vi "OutputDefault.vi"(6 "error in":errorcluster, 9 "Control Terminal in":refnum<class "ControlTerminal.lvclass">) -> (0 "error out":errorcluster, 3 "Control Terminal out":refnum<class "ControlTerminal.lvclass">, 4 "output default":string)   [LabVIEW 2014, in "ControlTerminal.lvclass"]
uses:
  ControlTerminal.lvclass
  Python/Parsing/Python Functions.lvlib
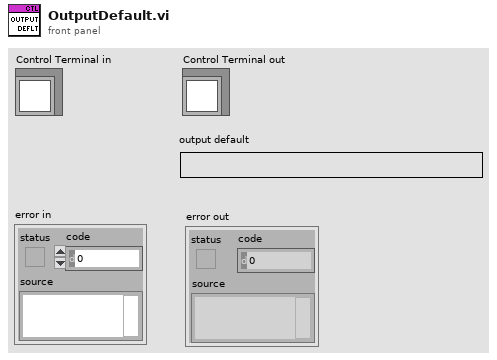
[diagram p1: front panel]
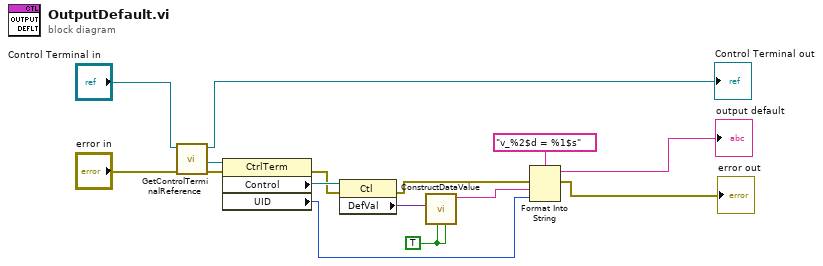
[diagram p0: block diagram]
diagram:
  w11 = TRUE ("value")
  n1 = call "GetControlTerminalReference.vi"("error in"="error in", "ControlTerminal in"="Control Terminal in") -> ("error out"=w5:errorcluster, "reference"=w4:refnum<vi>, "ControlTerminal out"=→"Control Terminal out":refnum<class "ControlTerminal.lvclass">)  [unwired: 7 in]
  n2 = property class="CtrlTerm"(reference=w4, error in=w5) -> (error out=w13:errorcluster, "Control"=w14:refnum<vi>, "UID"=w7:i32)  [unwired: 1 out]
  n3 = property class="Ctl"(reference=w14, error in=w13) -> (error out=w9:errorcluster, "DefVal"=w12:variant)  [unwired: 1 out]
  n4 = call "ConstructDataValue.vi"("label"=w11, "value"=w11, "Value"=w12) -> ("value"=w10:string)  [unwired: 6 in]
  n5 = Format Into String(format string="v_%2$d = %1$s", error in=w9, w10, w7) -> (resulting string=→"output default":string, error out=→"error out":errorcluster)  [unwired: 1 in]
